vi "Arrays_X8.vi"(0 "Array_CH3_IN":dbl[](array[numeric]), 1 "Array_CH4_IN":dbl[](array[numeric]), 2 "Array_CH5_IN":dbl[](array[numeric]), 3 "Array_CH6_IN":dbl[](array[numeric]), 4 "Array_CH7_IN":dbl[](array[numeric]), 5 "Array_CH8_IN":dbl[](array[numeric]), 6 "Datos_IN_X8":dbl[][](array[numeric]), 7 "Error In":errorcluster, 8 "Array_CH2_IN":dbl[](array[numeric]), 10 "Array_CH1_IN":dbl[](array[numeric])) -> (16 "Array_CH1_OUT":dbl[](array[numeric]), 18 "Array_CH2_OUT":dbl[](array[numeric]), 20 "Array_CH3_OUT":dbl[](array[numeric]), 21 "Array_CH4_OUT":dbl[](array[numeric]), 22 "Array_CH5_OUT":dbl[](array[numeric]), 23 "Array_CH6_OUT":dbl[](array[numeric]), 24 "Array_CH7_OUT":dbl[](array[numeric]), 25 "Array_CH8_OUT":dbl[](array[numeric]), 27 "Error Out":errorcluster)   [LabVIEW 2013]
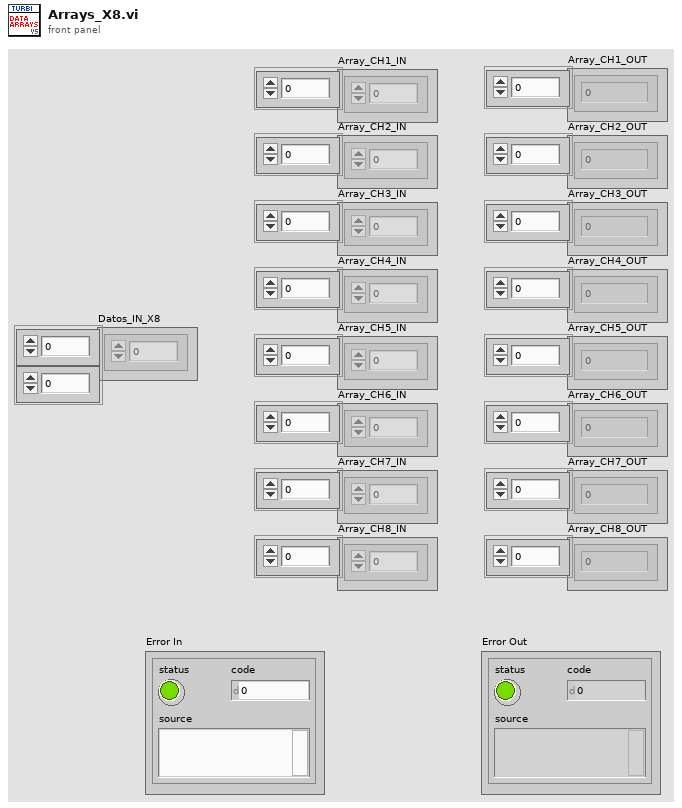
[diagram p1: front panel]
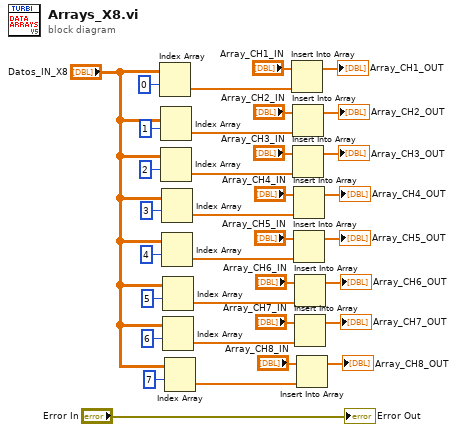
[diagram p0: block diagram]
diagram:
  n1 = Index Array(array="Datos_IN_X8", index (row)=0) -> (element=w33:dbl[])  [unwired: 1 in]
  n2 = Index Array(array="Datos_IN_X8", index (row)=1) -> (element=w28:dbl[])  [unwired: 1 in]
  n3 = Index Array(array="Datos_IN_X8", index (row)=2) -> (element=w25:dbl[])  [unwired: 1 in]
  n4 = Index Array(array="Datos_IN_X8", index (row)=3) -> (element=w20:dbl[])  [unwired: 1 in]
  n5 = Index Array(array="Datos_IN_X8", index (row)=4) -> (element=w17:dbl[])  [unwired: 1 in]
  n6 = Index Array(array="Datos_IN_X8", index (row)=5) -> (element=w12:dbl[])  [unwired: 1 in]
  n7 = Index Array(array="Datos_IN_X8", index (row)=6) -> (element=w9:dbl[])  [unwired: 1 in]
  n8 = Index Array(array="Datos_IN_X8", index (row)=7) -> (element=w4:dbl[])  [unwired: 1 in]
  n9 = Insert Into Array(array="Array_CH1_IN", new element=w33) -> (→"Array_CH1_OUT":dbl[])  [unwired: 1 in]
  n10 = Insert Into Array(array="Array_CH2_IN", new element=w28) -> (→"Array_CH2_OUT":dbl[])  [unwired: 1 in]
  n11 = Insert Into Array(array="Array_CH3_IN", new element=w25) -> (→"Array_CH3_OUT":dbl[])  [unwired: 1 in]
  n12 = Insert Into Array(array="Array_CH4_IN", new element=w20) -> (→"Array_CH4_OUT":dbl[])  [unwired: 1 in]
  n13 = Insert Into Array(array="Array_CH5_IN", new element=w17) -> (→"Array_CH5_OUT":dbl[])  [unwired: 1 in]
  n14 = Insert Into Array(array="Array_CH6_IN", new element=w12) -> (→"Array_CH6_OUT":dbl[])  [unwired: 1 in]
  n15 = Insert Into Array(array="Array_CH7_IN", new element=w9) -> (→"Array_CH7_OUT":dbl[])  [unwired: 1 in]
  n16 = Insert Into Array(array="Array_CH8_IN", new element=w4) -> (→"Array_CH8_OUT":dbl[])  [unwired: 1 in]
  "Error Out" <- "Error In"
